vi "Format Text Span.vi"(8 "Error in":errorcluster caption="Error in (no error)", 9 "Text Color (Unchanged)":u32(colorbox), 10 "BG Color (Unchanged)":u32(colorbox), 11 "Text":string) -> (0 "Error out":errorcluster, 3 "Formatted Span":string)   [LabVIEW 2023, in "Confluence Formatting.lvlib"]
uses:
  Confluence Formatting.lvlib
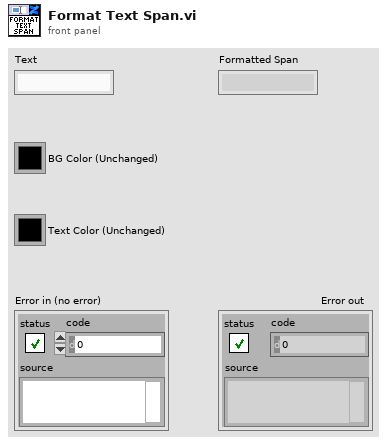
[diagram p1: front panel]
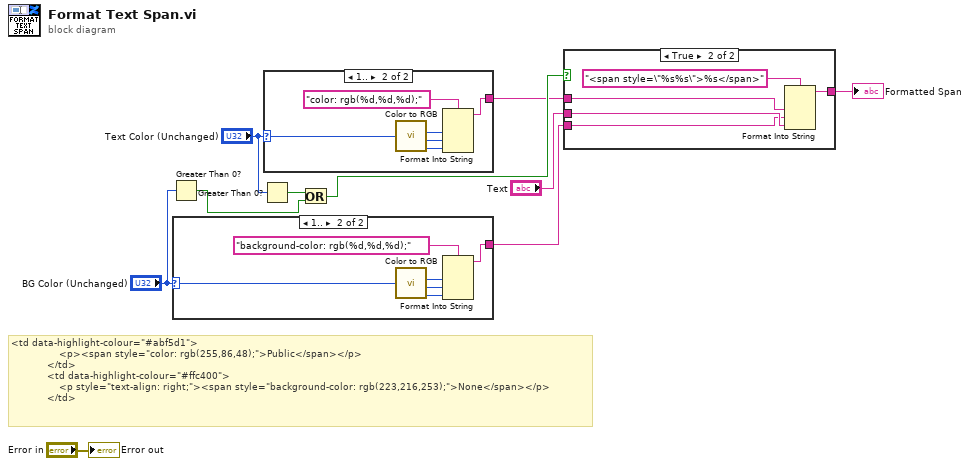
[diagram p0: block diagram]
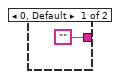
[diagram p3: hidden frame]
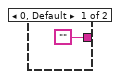
[diagram p4: hidden frame]
diagram:
  # "<td data-highlight-colour=\"#abf5d1\">\n                <p><span style=\"color: rgb(255,86,48);\">Public</span></p>\n            </td>\n            <td data-highlight-colour=\"#ffc400\">\n                <p style=\"text-align: right;\"><span style=\"background-color: rgb(223,216,253);\">None</span></p>\n            </td>"
  n1 = Greater Than 0?(x="BG Color (Unchanged)") -> (x > 0?=w9:bool)
  n2 = case shown="1.." "BG Color (Unchanged)" {
    selector: "BG Color (Unchanged)" -> [_ w16]
    tunnel: ["" w12] -> w4
    frame 0, Default {
    }
    frame 1.. {
      n3 = call <vilib>:"Color to RGB.vi"("Color"=w16) -> ("R"=w15:u8, "G"=w14:u8, "B"=w13:u8)  [unwired: 1 out]
      n4 = Format Into String(format string="background-color: rgb(%d,%d,%d);", w15, w14, w13) -> (resulting string=w12:string)  [unwired: 2 in, 1 out]
    }
  }
  n5 = Greater Than 0?(x="Text Color (Unchanged)") -> (x > 0?=w10:bool)
  n6 = case shown="1.." "Text Color (Unchanged)" {
    selector: "Text Color (Unchanged)" -> [_ w23]
    tunnel: ["" w19] -> w5
    frame 0, Default {
    }
    frame 1.. {
      n7 = call <vilib>:"Color to RGB.vi"("Color"=w23) -> ("R"=w22:u8, "G"=w21:u8, "B"=w20:u8)  [unwired: 1 out]
      n8 = Format Into String(format string="color: rgb(%d,%d,%d);", w22, w21, w20) -> (resulting string=w19:string)  [unwired: 2 in, 1 out]
    }
  }
  n9 = Or(x=w10, y=w9) -> (x .or. y?=w8:bool)
  n10 = case shown="True" w8 {
    tunnel: [w25 w29] -> w7
    tunnel: "Text" -> [w25 w28]
    tunnel: w5 -> [_ w27]
    tunnel: w4 -> [_ w26]
    frame False {
    }
    frame True {
      n11 = Format Into String(format string="<span style=\"%s%s\">%s</span>", w27, w26, w28) -> (resulting string=w29:string)  [unwired: 2 in, 1 out]
    }
  }
  "Formatted Span" <- w7
  "Error out" <- "Error in"
